vi "Determine Condition.vi"(8 "error in (no error)":errorcluster, 10 "RPM":dbl, 11 "RMS":dbl) -> (0 "error out":errorcluster, 3 "Condition":i32)   [LabVIEW 2026, in "Acquisition.lvlib"]
uses:
  Acquisition.lvlib
  Controls/Machine Speed.ctl
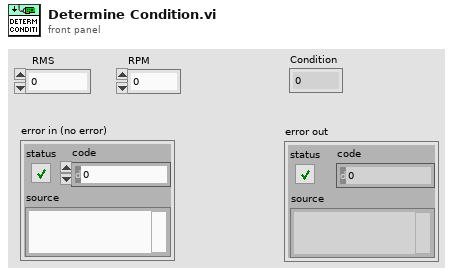
[diagram p1: front panel]
types:
  T1 = typedef "Machine Speed.ctl" = enum16{"Low Speed", "Medium Speed", "High Speed"}
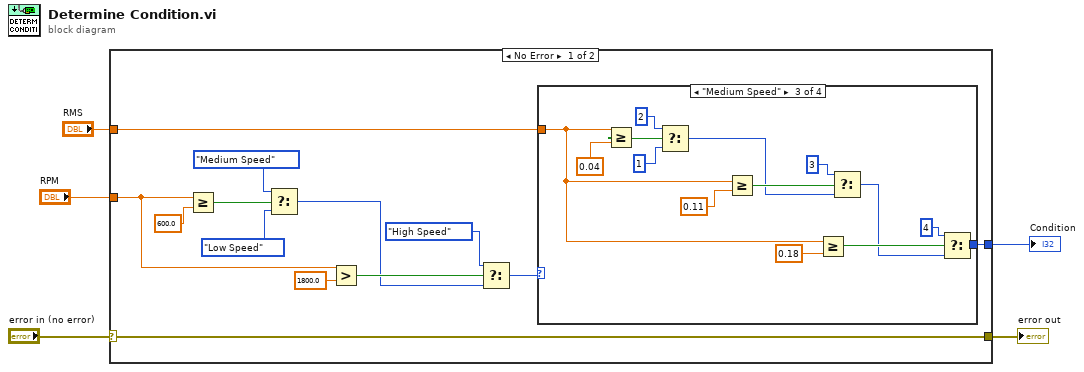
[diagram p0: block diagram]
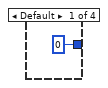
[diagram p2: hidden frame]
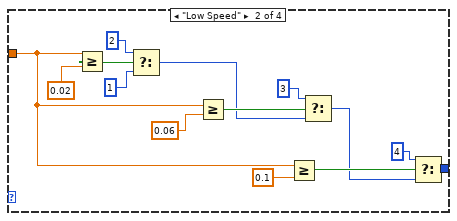
[diagram p3: hidden frame]
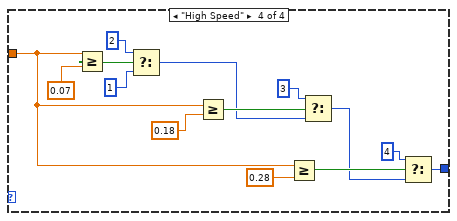
[diagram p4: hidden frame]
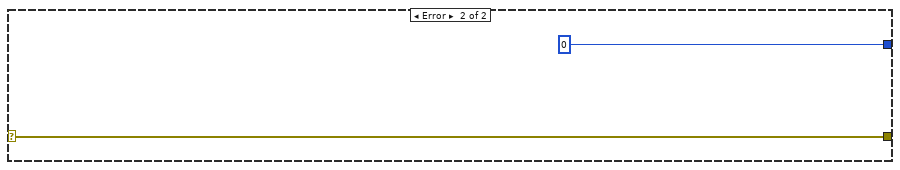
[diagram p5: hidden frame]
diagram:
  n1 = case shown="No Error" "error in (no error)" {
    selector: "error in (no error)" -> [w16 w63]
    tunnel: "RMS" -> [w18 _]
    tunnel: [w17 0] -> w2
    tunnel: [w16 w63] -> w3
    tunnel: "RPM" -> [w10 _]
    frame No Error {
      n2 = Greater Or Equal?(x=w10, y=600.0) -> (x >= y?=w15:bool)
      n3 = Select(t=Machine_Speed."Medium Speed", s=w15, f=Machine_Speed."Low Speed") -> (s? t:f=w7:T1)
      n4 = Greater?(x=w10, y=1800.0) -> (0:w9:bool)
      n5 = Select(t=Machine_Speed."High Speed", s=w9, f=w7) -> (s? t:f=w6:T1)
      n6 = case shown="\"Medium Speed\"" w6 {
        tunnel: w18 -> [_ w28 w42 w56]
        tunnel: [0 w24 w38 w52] -> w17
        frame Default {
        }
        frame "Low Speed" {
          n7 = Greater Or Equal?(x=w28, y=0.02 ("x")) -> (x >= y?=w33:bool)
          n8 = Select(t=2, s=w33, f=1) -> (s? t:f=w30:i32)
          n9 = Greater Or Equal?(x=w28, y=0.06 ("x")) -> (x >= y?=w32:bool)
          n10 = Greater Or Equal?(x=w28, y=0.1 ("x")) -> (x >= y?=w26:bool)
          n11 = Select(t=3, s=w32, f=w30) -> (s? t:f=w25:i32)
          n12 = Select(t=4, s=w26, f=w25) -> (s? t:f=w24:i32)
        }
        frame "Medium Speed" {
          n13 = Greater Or Equal?(x=w42, y=0.04 ("x")) -> (x >= y?=w47:bool)
          n14 = Select(t=2, s=w47, f=1) -> (s? t:f=w44:i32)
          n15 = Greater Or Equal?(x=w42, y=0.11 ("x")) -> (x >= y?=w46:bool)
          n16 = Greater Or Equal?(x=w42, y=0.18 ("x")) -> (x >= y?=w40:bool)
          n17 = Select(t=3, s=w46, f=w44) -> (s? t:f=w39:i32)
          n18 = Select(t=4, s=w40, f=w39) -> (s? t:f=w38:i32)
        }
        frame "High Speed" {
          n19 = Greater Or Equal?(x=w56, y=0.07 ("x")) -> (x >= y?=w61:bool)
          n20 = Select(t=2, s=w61, f=1) -> (s? t:f=w58:i32)
          n21 = Greater Or Equal?(x=w56, y=0.18 ("x")) -> (x >= y?=w60:bool)
          n22 = Greater Or Equal?(x=w56, y=0.28 ("x")) -> (x >= y?=w54:bool)
          n23 = Select(t=3, s=w60, f=w58) -> (s? t:f=w53:i32)
          n24 = Select(t=4, s=w54, f=w53) -> (s? t:f=w52:i32)
        }
      }
    }
    frame Error {
    }
  }
  "error out" <- w3
  "Condition" <- w2
